vi "I Exist.vi"(8 "error in (no error)":errorcluster, 11 "Guardian in":refnum<class "Guardian.lvclass">) -> (0 "error out":errorcluster, 3 "Guardian out":refnum<class "Guardian.lvclass">)   [LabVIEW 2026, in "TALOS.lvlib" / "Guardian.lvlib" / "Guardian.lvclass"]
uses:
  Guardian.lvclass
  C:/LabVIEW Code/TALOS/talos/Ancestor/Ancestor/Ancestor.lvclass
  Ancestor/Ancestor/Ancestor.lvclass/Ancestor.ctl
  Guardian.lvclass/Guardian.ctl
  Classes/Guardian List/Guardian List.lvclass
  Ancestor/Ancestor/Ancestor.lvclass
  TALOS.lvlib
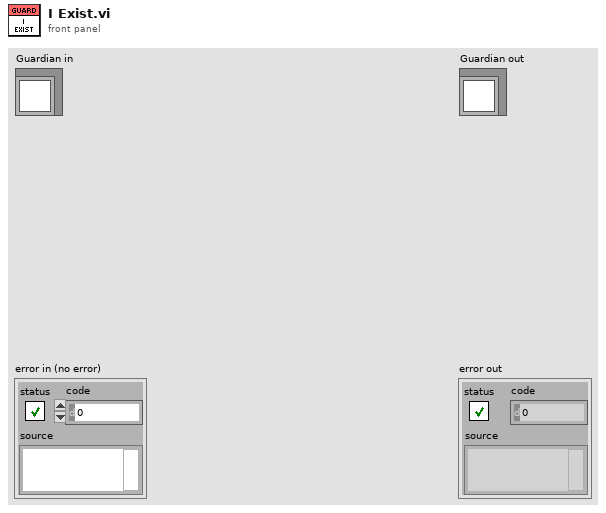
[diagram p1: front panel]
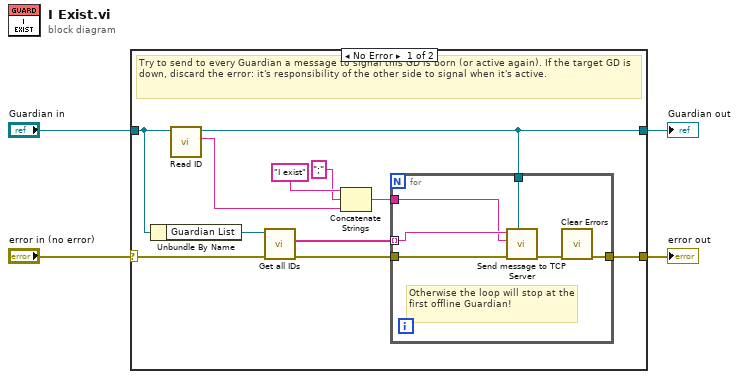
[diagram p0: block diagram]
diagram:
  n1 = case shown="No Error" "error in (no error)" {
    selector: "error in (no error)" -> [w11 w23]
    tunnel: [w8 w23] -> w3
    tunnel: [w7 w22] -> w1
    tunnel: "Guardian in" -> [w9 w22]
    frame No Error {
      # "Try to send to every Guardian a message to signal this GD is born (or active again). If the target GD is down, discard the error: it's responsibility of the other side to signal when it's active."
      n2 = Unbundle By Name(w9) -> ("Guardian List"=w14:refnum<class "Guardian List.lvclass">)
      n3 = call "Read ID.vi"("Ancestor in"=w9) -> ("ID"=w15:string, "Ancestor out"=w7:refnum<class "Guardian.lvclass">)  [unwired: 8 in, 1 out]
      n4 = call-dynamic "Get all IDs.vi"("error in (no error)"=w11, "Guardian List in"=w14) -> ("error out"=w12:errorcluster, "All IDs"=w13:string[])  [unwired: 7 in, 1 out]
      n5 = Concatenate Strings("I exist" ("Message"), ";" ("string"), w15) -> (w5:string)
      n6 = for {
        tunnel: w12 -> [w21]
        tunnel: [w17] -> w8
        tunnel: w13 -> [w20] mode=indexing
        tunnel: w5 -> [w16]
        tunnel: w7 -> [w18]
        # "Otherwise the loop will stop at the first offline Guardian!"
        n7 = call "Send message to TCP Server.vi"("LabVIEW Object"=w18, "error in (no error)"=w21, "String"=w16, "Guardian ID"=w20) -> ("error out"=w19:errorcluster)  [unwired: 7 in]
        n8 = call <vilib>:"Clear Errors.vi"("error in (no error)"=w19) -> ("error out"=w17:errorcluster)  [unwired: 5 in, 1 out]
      }
    }
    frame Error {
    }
  }
  "error out" <- w3
  "Guardian out" <- w1
